vi "Setup.vi"(6 "Number of Gate":u16=1, 8 "error in (no error)":errorcluster, 9 "Transfer Mode":T1=2 items=["Single"=1, "Block"=2], 10 "Gate Time":T2=6 items=["50u"=2, "100u"=3, "200u"=4, "500u"=5, "1m"=6, "2m"=7, "5m"=8, "10m"=9, "20m"=10, "50m"=11, "100m"=12, "200m"=13, "500m"=14, "1"=15, "2"=16, "5"=17, "10"=18], 11 "Handle":u32) -> (0 "error out":errorcluster, 3 "Handle out":u32)   [LabVIEW 2016, in "Photon Counter.lvlib" / "C8855-01.lvlib"]
doc: "BOOL C8855API __stdcall C8855Setup( HANDLE hC8855,\n BYTE GateTime,\n BYTE TransferMode,\n WORD NumberOfGate);"
uses:
  C8855-01.lvlib
  Gate Time.ctl
  Transfer Mode.ctl
  C8855-01api.dll
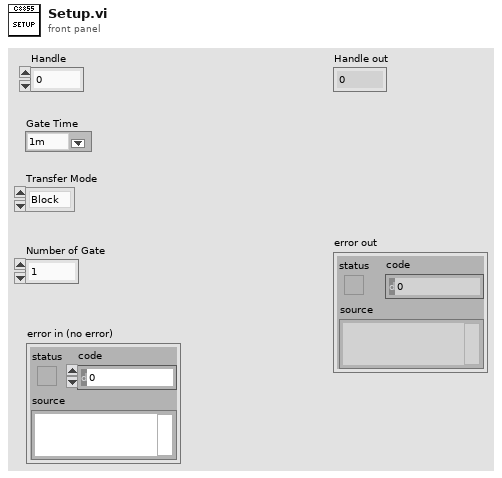
[diagram p1: front panel]
types:
  T1 = typedef "Photon Counter.lvlib/C8855-01.lvlib/Transfer Mode.ctl" = u8
  T2 = typedef "Photon Counter.lvlib/C8855-01.lvlib/Gate Time.ctl" = u8
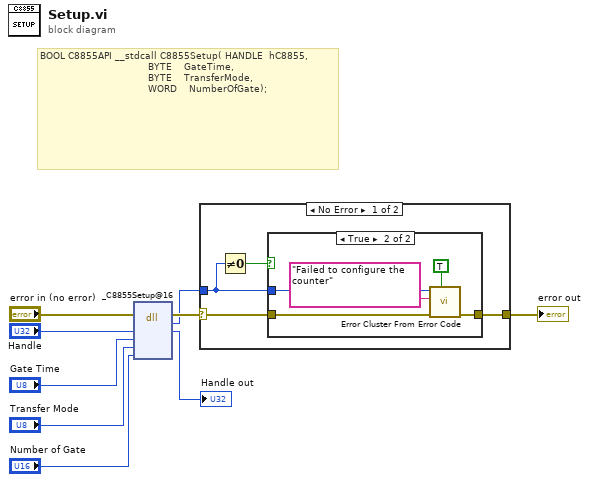
[diagram p0: block diagram]
diagram:
  # "BOOL C8855API __stdcall C8855Setup( HANDLE  hC8855,\n                                    BYTE    GateTime,\n                                    BYTE    TransferMode,\n                                    WORD    NumberOfGate);"
  n1 = dll-call lib="Z:/VM Shared Folder/Trace Grabber/Drivers/C8855-01/C8855-01api.*" fn="_C8855Setup@16"(error in="error in (no error)", "Handle"="Handle", "Gate Time"="Gate Time", "Transfer Mode"="Transfer Mode", "Number of Gate"="Number of Gate") -> (error out=w3:errorcluster, "return type"=w2:i32, "Handle"=→"Handle out":u32)  [unwired: 5 in, 1 out]
  n2 = case shown="No Error" w3 {
    selector: w3 -> [w12 w20]
    tunnel: w2 -> [w10 _]
    tunnel: [w11 w20] -> w1
    frame No Error {
      n3 = Not Equal To 0?(x=w10) -> (x != 0?=w13:bool)
      n4 = case shown="True" w13 {
        tunnel: w12 -> [w14 w18]
        tunnel: [w14 w17] -> w11
        tunnel: w10 -> [_ w16]
        frame False {
        }
        frame True {
          n5 = call <vilib>:"Error Cluster From Error Code.vi"("show call chain? (False)"=TRUE, "error in (no error)"=w18, "error message (\"\")"="Failed to configure the counter" ("error message (\"\")"), "error code (0)"=w16) -> ("error out"=w17:errorcluster)  [unwired: 5 in]
        }
      }
    }
    frame Error {
    }
  }
  "error out" <- w1
